vi "Read ECU String.vi"(8 "error in (no error)":errorcluster, 11 "String":string="1,HS,OK,35000,568,1.32,11,30.1") -> (0 "error out":errorcluster, 1 "Pump Voltage":dbl, 2 "Turbine Temp":dbl, 3 "Turbine RPM":dbl, 4 "Turbine State":string, 5 "Throttle Position":dbl)   [LabVIEW 2014]
panel:
  out "Turbine State":dbl
  # "1,HS,OK,35000,568,1.32,11,30.1"
  # "1,HS,OK,0,20,0,0,0"
  # "1,RAC,1\n1,HS,OK,0,20,0,0,0"
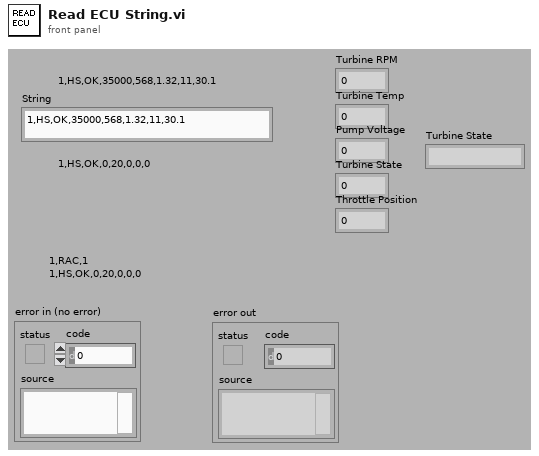
[diagram p1: front panel]
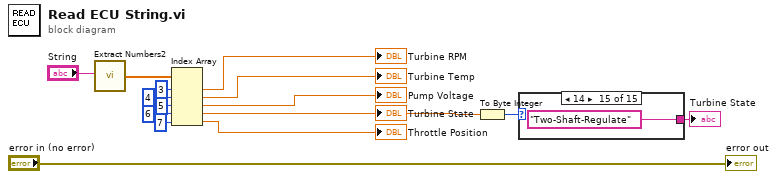
[diagram p0: block diagram]
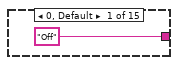
[diagram p2: hidden frame]
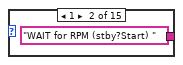
[diagram p3: hidden frame]
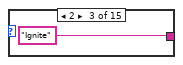
[diagram p4: hidden frame]
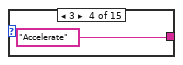
[diagram p5: hidden frame]
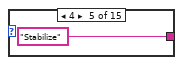
[diagram p6: hidden frame]
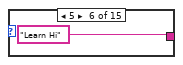
[diagram p7: hidden frame]
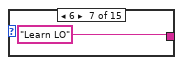
[diagram p8: hidden frame]
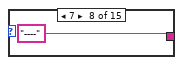
[diagram p9: hidden frame]
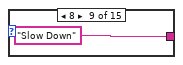
[diagram p10: hidden frame]
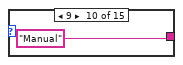
[diagram p11: hidden frame]
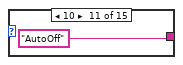
[diagram p12: hidden frame]
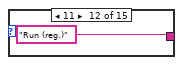
[diagram p13: hidden frame]
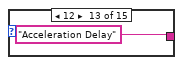
[diagram p14: hidden frame]
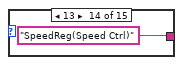
[diagram p15: hidden frame]
diagram:
  n1 = call "Extract Numbers2.vi"("String"="String") -> ("Output Array"=w2:dbl[])  [unwired: 4 out]
  n2 = Index Array(array=w2, index #1=3 ("index"), index #2=4 ("index"), index #3=5 ("index"), index #4=6 ("index"), index #5=7 ("index")) -> (element #1=→"Turbine RPM":dbl, element #2=→"Turbine Temp":dbl, element #3=→"Pump Voltage":dbl, element #4=w6:dbl, element #5=→"Throttle Position":dbl)
  "Turbine State" <- w6
  n3 = To Byte Integer(number=w6) -> (8bit integer=w5:i8)
  n4 = case shown="14" w5 {
    tunnel: ["Off" "WAIT for RPM (stby?Start) " "Ignite" "Accelerate" "Stabilize" "Learn Hi" "Learn LO" "----" "Slow Down" "Manual" "AutoOff" "Run (reg.)" "Acceleration Delay" "SpeedReg(Speed Ctrl)" "Two-Shaft-Regulate"] -> w4
    frame 0, Default {
    }
    frame 1 {
    }
    frame 2 {
    }
    frame 3 {
    }
    frame 4 {
    }
    frame 5 {
    }
    frame 6 {
    }
    frame 7 {
    }
    frame 8 {
    }
    frame 9 {
    }
    frame 10 {
    }
    frame 11 {
    }
    frame 12 {
    }
    frame 13 {
    }
    frame 14 {
    }
  }
  "Turbine State" <- w4
  "error out" <- "error in (no error)"
